vi "SG Initialize - TOI.vi"(8 "error in (no error)":errorcluster, 11 "RFSG Settings":T1 {"Attenuation"."Attenuation"."s2p File"."RFSG S-parameters Orientation" items=["Port1 Towards DUT"=24000, "Port2 Towards DUT"=24001]; "Attenuation"."Attenuation"."Contant Attenuation"."RFSG External Attenuation (dB)" format="%.2f"; "IQ Rate (S/sec)" format="%#.3p"}) -> (0 "error out":errorcluster, 3 "RFSG Session Out":refnum<k15>)   [LabVIEW 2023]
uses:
  Controls/RFSG Config - TOI.ctl
  FPT Shared VIs/De-embedding/RFsg Config.ctl
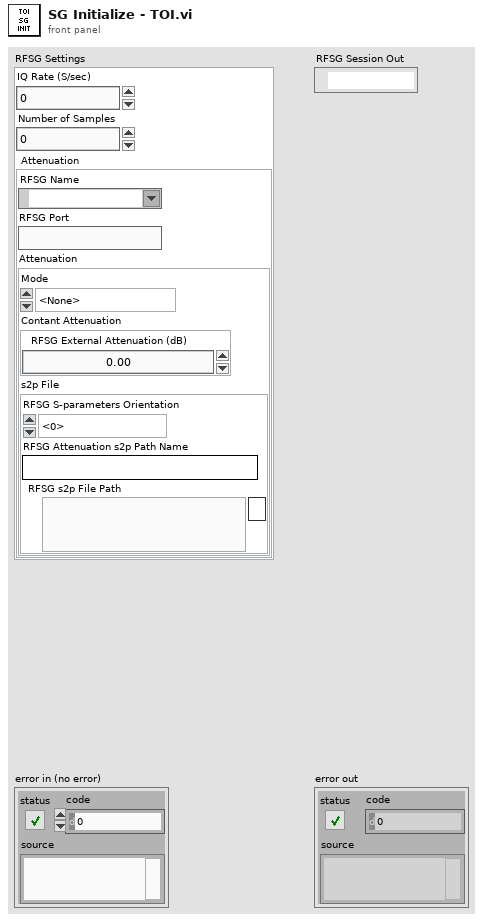
[diagram p1: front panel]
types:
  T1 = typedef "RFSG Config - TOI.ctl" = cluster{"IQ Rate (S/sec)":dbl, "Number of Samples":i32, "Attenuation":T2}
  T2 = typedef "RFsg Config.ctl" = cluster{"RFSG Name":refnum<k15>, "RFSG Port":string, "Attenuation":cluster{"Mode":enum32{"<None>", "Constant Attenuation", "s2p File"}, "Contant Attenuation":cluster{"RFSG External Attenuation (dB)":dbl}, "s2p File":cluster{"RFSG S-parameters Orientation":i32, "RFSG Attenuation s2p Path Name":string, "RFSG s2p File Path":path}}}
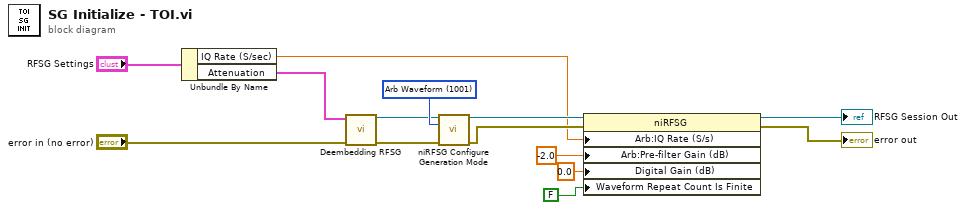
[diagram p0: block diagram]
diagram:
  w13 = 1001 items=["CW"=1000, "Arb Waveform"=1001, "Script"=1002] ("generation mode")
  n1 = Unbundle By Name("RFSG Settings") -> ("IQ Rate (S/sec)"=w1:dbl, "Attenuation"=w2:T2)
  n2 = call "Deembedding RFSG.vi"("error in"="error in (no error)", "RFSG Settings"=w2) -> ("error out"=w7:errorcluster, "IVI Refnum out"=w4:refnum<k15>)  [unwired: 8 in]
  n3 = call <instrlib>:"niRFSG Configure Generation Mode.vi"("instrument handle"=w4, "generation mode"=w13, "error in"=w7) -> ("instrument handle out"=w5:refnum<k15>, "error out"=w6:errorcluster)  [unwired: 11 in]
  n4 = property class="niRFSG"(reference=w5, error in=w6, "Arb:IQ Rate (S/s)"=w1, "Arb:Pre-filter Gain (dB)"=-2.0 ("RF:Advanced:AWG:DUC Pre-filter Gain (dB)"), "Digital Gain (dB)"=0.0 ("Arb:Advanced:Digital Gain (dB)"), "Waveform Repeat Count Is Finite"=FALSE ("Arb:Waveform Repeat Count Is Finite")) -> (reference out=→"RFSG Session Out":refnum<k15>, error out=→"error out":errorcluster)
